vi "Destroy.vi"(0 "reference in":refnum<class "UE_master.lvclass">, 5 "error in (no error)":errorcluster) -> (14 "reference out":refnum<class "UE_master.lvclass">, 19 "error out":errorcluster)   [LabVIEW 2019, in "CommandResponse communication.lvlib" / "UE_master.lvclass"]
doc: "Destructor."
uses:
  UE_master.lvclass
  CR_master_class/CR_master.lvclass
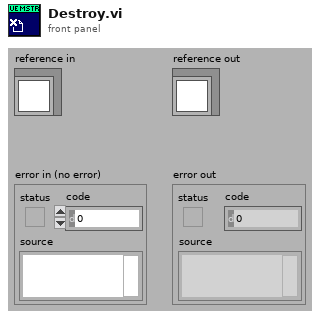
[diagram p1: front panel]
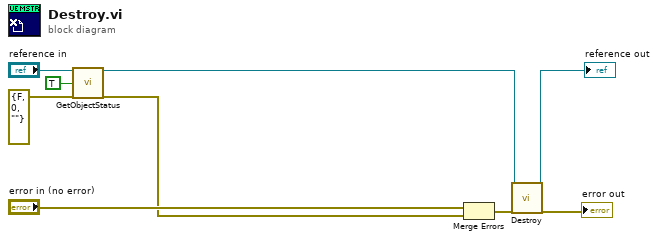
[diagram p0: block diagram]
diagram:
  n1 = call-dynamic "GetObjectStatus.vi"("reference in"="reference in", "simple info (F)"=TRUE ("simple info"), "error in (no error)"=errorcluster {"status"=FALSE, "code"=0, "source"=""}) -> ("reference out"=w1:refnum<class "UE_master.lvclass">, "error out"=w2:errorcluster)  [unwired: 5 in, 10 out]
  n2 = Merge Errors("error in (no error)", w2) -> (w8:errorcluster)
  n3 = call-parent "Destroy.vi"("reference in"=w1, "error in (no error)"=w8) -> ("reference out"=→"reference out":refnum<class "UE_master.lvclass">, "error out"=→"error out":errorcluster)  [unwired: 16 in]
